vi "Actor Core.vi"(8 "error in":errorcluster, 11 "Focus Indicator in":refnum<class "Focus Indicator.lvclass">) -> (0 "error out":errorcluster, 3 "Actor out":refnum<class "Actor.lvclass">)   [LabVIEW 2015, in "Focus Indicator.lvlib" / "Focus Indicator.lvclass"]
doc: "(<B>Filename</B>: Actor Framework.lvlib:Actor.lvclass:Actor Core.vi)\n\nReceives messages to the actor, reacts to them, and initiates any error handling that may shut the actor down.\n\nDescendant classes may override this VI to append parallel tasks for the actor to complete while it handles messages. Overrides use the Call Parent Method node."
uses:
  Focus Indicator.lvclass
  UI Window/UI Window.lvclass
  Resources/GLOBAL/GLOBAL Time-critical.vi
  <vilib>/Analysis/NI_AALPro.lvlib
  <vilib>/Analysis/2dsp.llb/Real FFT.vi
  <vilib>/ActorFramework/Actor/Actor.lvclass
panel:
  in  "Stop Button":bool
  out "Focus Chart":cluster{dbl, dbl}(graph)
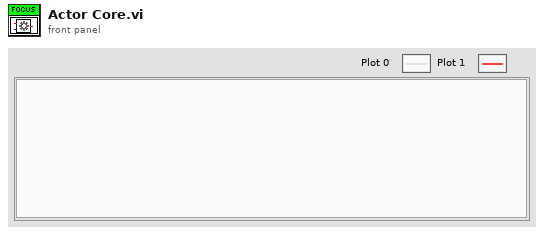
[diagram p1: front panel]
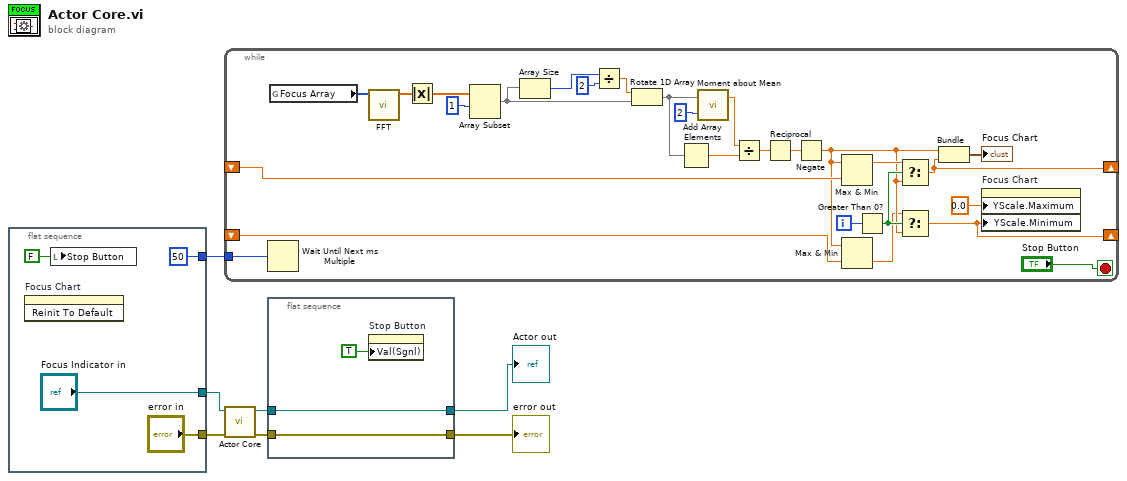
[diagram p0: block diagram]
diagram:
  n1 = flat-sequence {
    tunnel: ["error in"] -> w7
    tunnel: ["Focus Indicator in"] -> w6
    tunnel: [u32 50 ("millisecond multiple")] -> w1
    frame #0 {
      n2 = invoke on="Focus Chart" class="WFChart (strict)" method="Reinit To Default"() -> ()  [unwired: 3 in, 3 out]
      n3 = local write "Stop Button"(FALSE ("Stop Button")) -> ()
    }
  }
  n4 = while {
    tunnel: w1 -> [w37]
    shift-right: [w19] -> _
    shift-left: _ -> [w27]
    shift-right: [w15] -> _
    shift-left: _ -> [w13]
    i -> [w24]
    stop <- "Stop Button" stop-if-true
    n5 = Wait Until Next ms Multiple(millisecond multiple=w37) -> ()  [unwired: 1 out]
    n6 = global read "GLOBAL Time-critical.vi" "Focus Array"() -> (w33:u16[])
    n7 = call-poly <vilib>:"FFT.vi"("X"=w33) -> ("FFT {X}"=w35:cdb[])  [unwired: 9 in, 1 out]
    n8 = Absolute Value(x=w35) -> (abs(x)=w28:dbl[])
    n9 = Array Subset(array=w28, index=1) -> (w29:dbl[])  [unwired: 1 in]
    n10 = Array Size(array=w29) -> (size(s)=w32:i32)
    n11 = Divide(x=w32, y=2) -> (x/y=w30:dbl)
    n12 = Rotate 1D Array(1:w29, 2:w30) -> (0:w26:dbl[])
    n13 = Add Array Elements(numeric array=w26) -> (sum=w25:dbl)
    n14 = call <vilib>:"Moment about Mean.vi"("order"=2, "X"=w26) -> ("moment"=w23:dbl)  [unwired: 1 out]
    n15 = Divide(x=w23, y=w25) -> (x/y=w21:dbl)
    n16 = Reciprocal(x=w21) -> (1/x=w20:dbl)
    n17 = Negate(x=w20) -> (-x=w14:dbl)
    n18 = Max & Min(x=w14, y=w27) -> (max(x,y)=w17:dbl)  [unwired: 1 out]
    n19 = Max & Min(x=w14, y=w13) -> (min(x,y)=w12:dbl)  [unwired: 1 out]
    n20 = Greater Than 0?(x=w24) -> (x > 0?=w16:bool)
    n21 = Select(t=w17, s=w16, f=w14) -> (s? t:f=w19:dbl)
    n22 = Select(t=w12, s=w16, f=w14) -> (s? t:f=w15:dbl)
    n23 = Bundle(w14, w19) -> (→"Focus Chart":cluster{dbl, dbl})  [unwired: 1 in]
    n24 = property on="Focus Chart" class="WFChart (strict)"("YScale.Maximum"=0.0 ("Y Scale.Range:Minimum"), "YScale.Minimum"=w15) -> ()  [unwired: 2 in, 2 out]
  }
  n25 = call-parent "Actor Core.vi"("error in"=w7, "UI Window in"=w6) -> ("error out"=w5:errorcluster, "Actor out"=w3:refnum<class "Actor.lvclass">)  [unwired: 8 in]
  n26 = flat-sequence {
    tunnel: w5 -> [w41]
    tunnel: [w41] -> w4
    tunnel: w3 -> [w40]
    tunnel: [w40] -> w2
    frame #0 {
      n27 = property on="Stop Button" class="Bool (strict)"("Val(Sgnl)"=TRUE ("Value (Signaling)")) -> ()  [unwired: 2 in, 2 out]
    }
  }
  "error out" <- w4
  "Actor out" <- w2
